vi "Configure New Assert Display.vi"(8 "error in (no error)":errorcluster) -> (0 "error out":errorcluster, 3 "Assert Display out":refnum<class "Assert Display.lvclass">)   [LabVIEW 2016, in "Assert Display.lvlib" / "Assert Display.lvclass"]
uses:
  Assert Display.lvclass
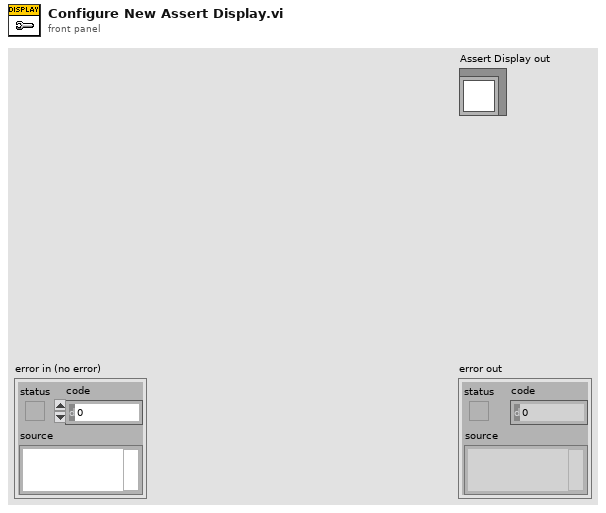
[diagram p1: front panel]
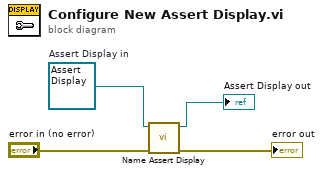
[diagram p0: block diagram]
diagram:
  w2 = refnum<class "Assert Display.lvclass"> refnum  # Assert Display in
  n1 = call "Name Assert Display.vi"("error in (no error)"="error in (no error)", "Assert Display in"=w2) -> ("error out"=→"error out":errorcluster, "Assert Display out"=→"Assert Display out":refnum<class "Assert Display.lvclass">)  [unwired: 8 in]
